vi "Get_System_Boolean_Values.vi"(2 "error in":errorcluster, 3 "Data in":T1) -> (0 "error out":errorcluster, 1 "Data out":T1)   [LabVIEW 2017]
uses:
  Type_Defs/Data.ctl
  Type_Defs/Diagnostics.ctl
  Type_Defs/Systems.ctl
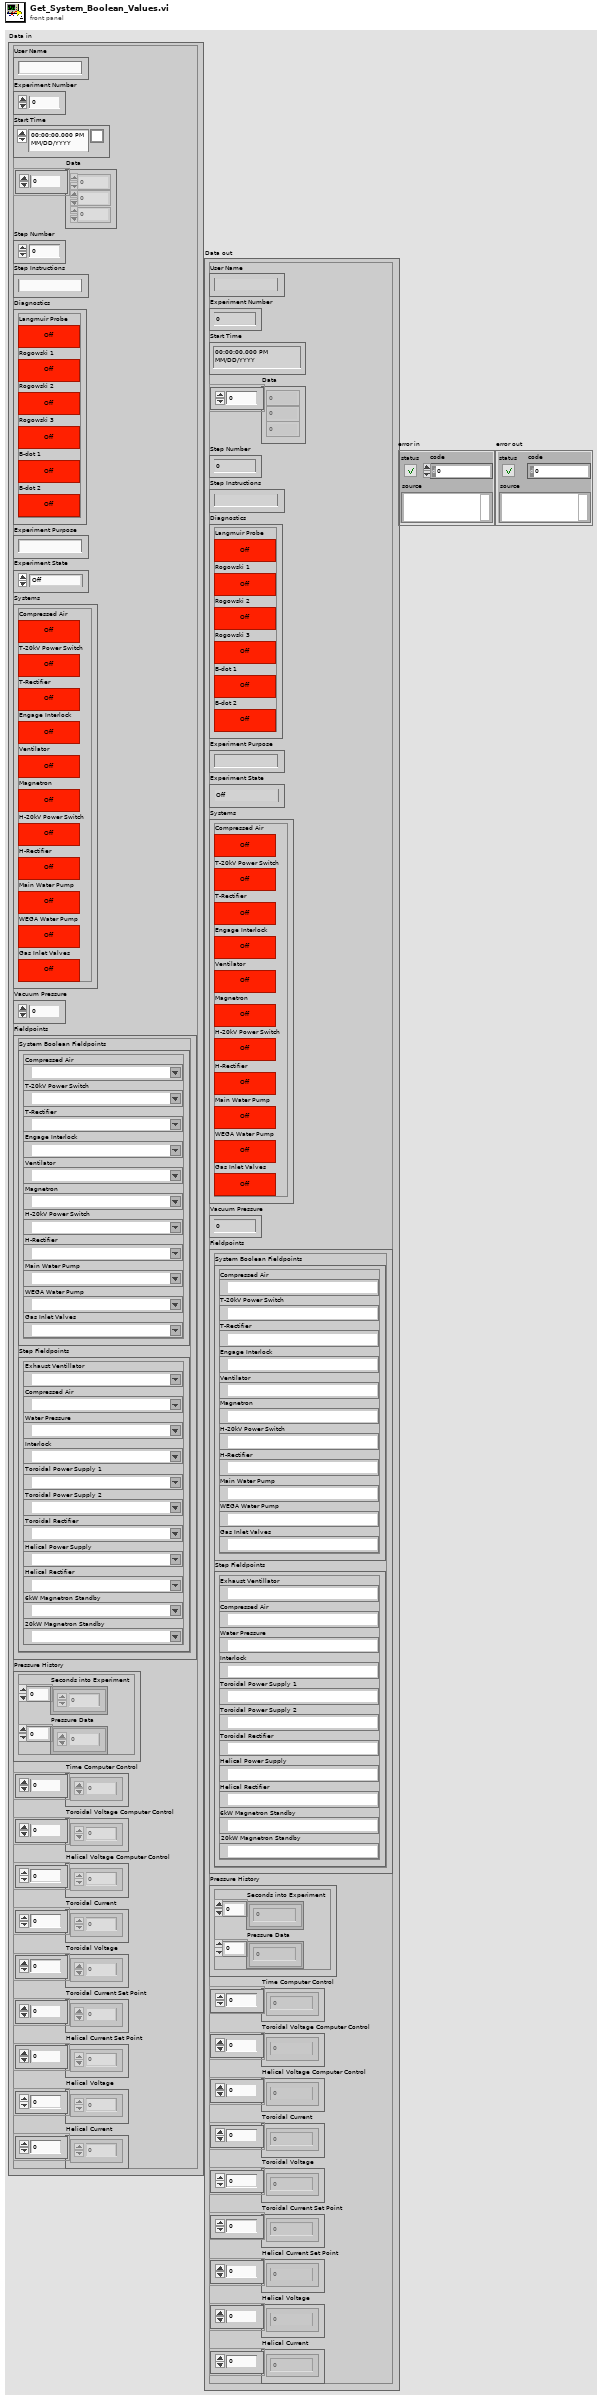
[diagram p1: front panel]
types:
  T1 = typedef "Data.ctl" = cluster{"User Name":string, "Experiment Number":i32, "Start Time":timestamp, "Data":dbl[], "Step Number":i32, "Step Instructions":string, "Diagnostics":T2, "Experiment Purpose":string, "Experiment State":enum16{"Off", "Setting Up", "Ready", "In Progress", "Shutting Down"}, "Systems":T3, "Vacuum Pressure":dbl, "Fieldpoints":cluster{"System Boolean Fieldpoints":cluster{"Compressed Air":refnum<k21>, "T-20kV Power Switch":refnum<k21>, "T-Rectifier":refnum<k21>, "Engage Interlock":refnum<k21>, "Ventilator":refnum<k21>, "Magnetron":refnum<k21>, "H-20kV Power Switch":refnum<k21>, "H-Rectifier":refnum<k21>, "Main Water Pump":refnum<k21>, "WEGA Water Pump":refnum<k21>, "Gas Inlet Valves":refnum<k21>}, "Step Fieldpoints":cluster{"Exhaust Ventillator":refnum<k21>, "Compressed Air":refnum<k21>, "Water Pressure":refnum<k21>, "Interlock":refnum<k21>, "Toroidal Power Supply 1":refnum<k21>, "Toroidal Power Supply 2":refnum<k21>, "Toroidal Rectifier":refnum<k21>, "Helical Power Supply":refnum<k21>, "Helical Rectifier":refnum<k21>, "6kW Magnetron Standby":refnum<k21>, "20kW Magnetron Standby":refnum<k21>}}, "Pressure History":cluster{"Seconds into Experiment":i32[], "Pressure Data":dbl[]}, "Time Computer Control":dbl[], "Toroidal Voltage Computer Control":dbl[], "Helical Voltage Computer Control":dbl[], "Toroidal Current":dbl[], "Toroidal Voltage":dbl[], "Toroidal Current Set Point":dbl[], "Helical Current Set Point":dbl[], "Helical Voltage":dbl[], "Helical Current":dbl[]}
  T2 = typedef "Diagnostics.ctl" = cluster{"Langmuir Probe":bool, "Rogowski 1":bool, "Rogowski 2":bool, "Rogowski 3":bool, "B-dot 1":bool, "B-dot 2":bool}
  T3 = typedef "Systems.ctl" = cluster{"Compressed Air":bool, "T-20kV Power Switch":bool, "T-Rectifier":bool, "Engage Interlock":bool, "Ventilator":bool, "Magnetron":bool, "H-20kV Power Switch":bool, "H-Rectifier":bool, "Main Water Pump":bool, "WEGA Water Pump":bool, "Gas Inlet Valves":bool}
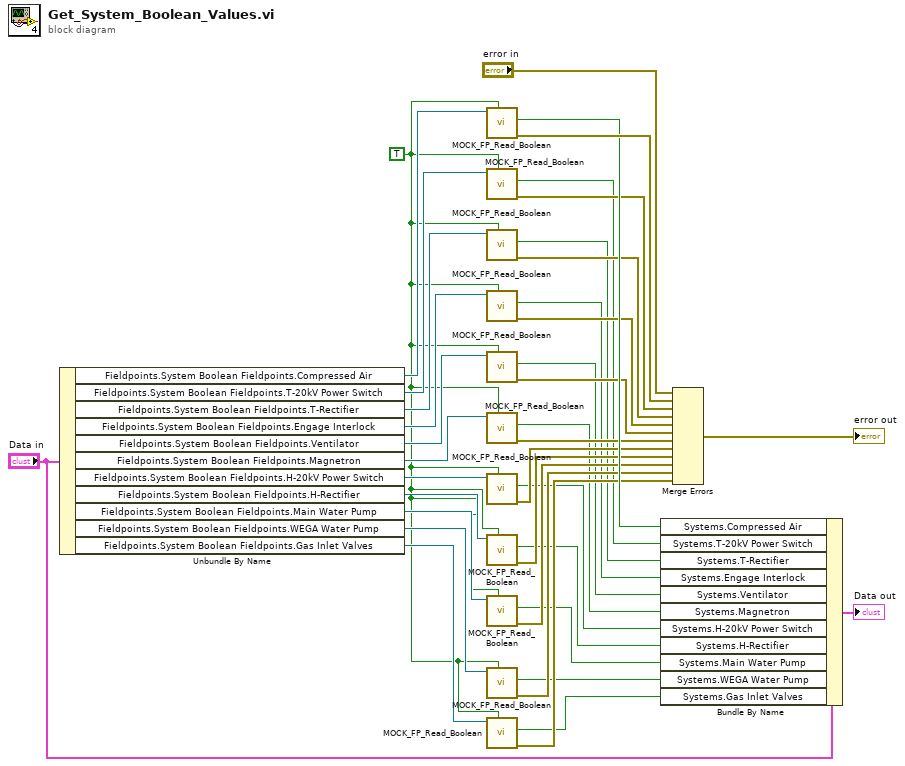
[diagram p0: block diagram]
diagram:
  w1 = TRUE ("Type")
  n1 = Unbundle By Name("Data in") -> ("Fieldpoints.System Boolean Fieldpoints.Compressed Air"=w38:refnum<k21>, "Fieldpoints.System Boolean Fieldpoints.T-20kV Power Switch"=w33:refnum<k21>, "Fieldpoints.System Boolean Fieldpoints.T-Rectifier"=w32:refnum<k21>, "Fieldpoints.System Boolean Fieldpoints.Engage Interlock"=w31:refnum<k21>, "Fieldpoints.System Boolean Fieldpoints.Ventilator"=w30:refnum<k21>, "Fieldpoints.System Boolean Fieldpoints.Magnetron"=w29:refnum<k21>, "Fieldpoints.System Boolean Fieldpoints.H-20kV Power Switch"=w28:refnum<k21>, "Fieldpoints.System Boolean Fieldpoints.H-Rectifier"=w27:refnum<k21>, "Fieldpoints.System Boolean Fieldpoints.Main Water Pump"=w26:refnum<k21>, "Fieldpoints.System Boolean Fieldpoints.WEGA Water Pump"=w25:refnum<k21>, "Fieldpoints.System Boolean Fieldpoints.Gas Inlet Valves"=w24:refnum<k21>)
  n2 = call "MOCK_FP_Read_Boolean.vi"("Type"=w1, "FieldPoint IO Point In"=w38) -> ("error out"=w35:errorcluster, "Boolean"=w34:bool)  [unwired: 6 in, 2 out]
  n3 = call "MOCK_FP_Read_Boolean.vi"("Type"=w1, "FieldPoint IO Point In"=w33) -> ("error out"=w23:errorcluster, "Boolean"=w12:bool)  [unwired: 6 in, 2 out]
  n4 = call "MOCK_FP_Read_Boolean.vi"("Type"=w1, "FieldPoint IO Point In"=w32) -> ("error out"=w22:errorcluster, "Boolean"=w11:bool)  [unwired: 6 in, 2 out]
  n5 = call "MOCK_FP_Read_Boolean.vi"("Type"=w1, "FieldPoint IO Point In"=w31) -> ("error out"=w21:errorcluster, "Boolean"=w10:bool)  [unwired: 6 in, 2 out]
  n6 = call "MOCK_FP_Read_Boolean.vi"("Type"=w1, "FieldPoint IO Point In"=w30) -> ("error out"=w20:errorcluster, "Boolean"=w9:bool)  [unwired: 6 in, 2 out]
  n7 = call "MOCK_FP_Read_Boolean.vi"("Type"=w1, "FieldPoint IO Point In"=w29) -> ("error out"=w19:errorcluster, "Boolean"=w8:bool)  [unwired: 6 in, 2 out]
  n8 = call "MOCK_FP_Read_Boolean.vi"("Type"=w1, "FieldPoint IO Point In"=w28) -> ("error out"=w18:errorcluster, "Boolean"=w6:bool)  [unwired: 6 in, 2 out]
  n9 = call "MOCK_FP_Read_Boolean.vi"("Type"=w1, "FieldPoint IO Point In"=w27) -> ("error out"=w17:errorcluster, "Boolean"=w5:bool)  [unwired: 6 in, 2 out]
  n10 = call "MOCK_FP_Read_Boolean.vi"("Type"=w1, "FieldPoint IO Point In"=w26) -> ("error out"=w16:errorcluster, "Boolean"=w4:bool)  [unwired: 6 in, 2 out]
  n11 = call "MOCK_FP_Read_Boolean.vi"("Type"=w1, "FieldPoint IO Point In"=w25) -> ("error out"=w15:errorcluster, "Boolean"=w3:bool)  [unwired: 6 in, 2 out]
  n12 = call "MOCK_FP_Read_Boolean.vi"("Type"=w1, "FieldPoint IO Point In"=w24) -> ("error out"=w14:errorcluster, "Boolean"=w2:bool)  [unwired: 6 in, 2 out]
  n13 = Bundle By Name(cluster="Data in", "Systems.Compressed Air"=w34, "Systems.T-20kV Power Switch"=w12, "Systems.T-Rectifier"=w11, "Systems.Engage Interlock"=w10, "Systems.Ventilator"=w9, "Systems.Magnetron"=w8, "Systems.H-20kV Power Switch"=w6, "Systems.H-Rectifier"=w5, "Systems.Main Water Pump"=w4, "Systems.WEGA Water Pump"=w3, "Systems.Gas Inlet Valves"=w2) -> (→"Data out":T1)
  n14 = Merge Errors("error in", w35, w23, w22, w21, w20, w19, w18, w17, w16, w15, w14) -> (→"error out":errorcluster)
